vi "ti2.vi"() -> ()   [LabVIEW 2010]
uses:
  typedefs/inspector_state_enum.ctl
  <vilib>/Utility/file.llb/Read From Spreadsheet File (DBL).vi
panel:
  in  "Filter pixels":i32=1 min=1 max=10000 step=1
  in  "Postprocessing":enum32{"Unfiltered", "Filtered"}(radio)
  in  "Channel selection":enum32{"Channel 1", "Channel 2", "Channel 3"}(radio)
  out "Current file":path
  out "Loading":bool
  in  "file path":path
  in  "ZoomOut":bool
  in  "ZoomIn":bool
  in  "Quit":bool
  in  "Load":bool
  out "Overview Graph":cluster{dbl, dbl, "Data out":dbl[]}(graph)
  out "Analysis Graph":dbl[](graph)
  # "Fiber - fMRI\nTrace inspector"
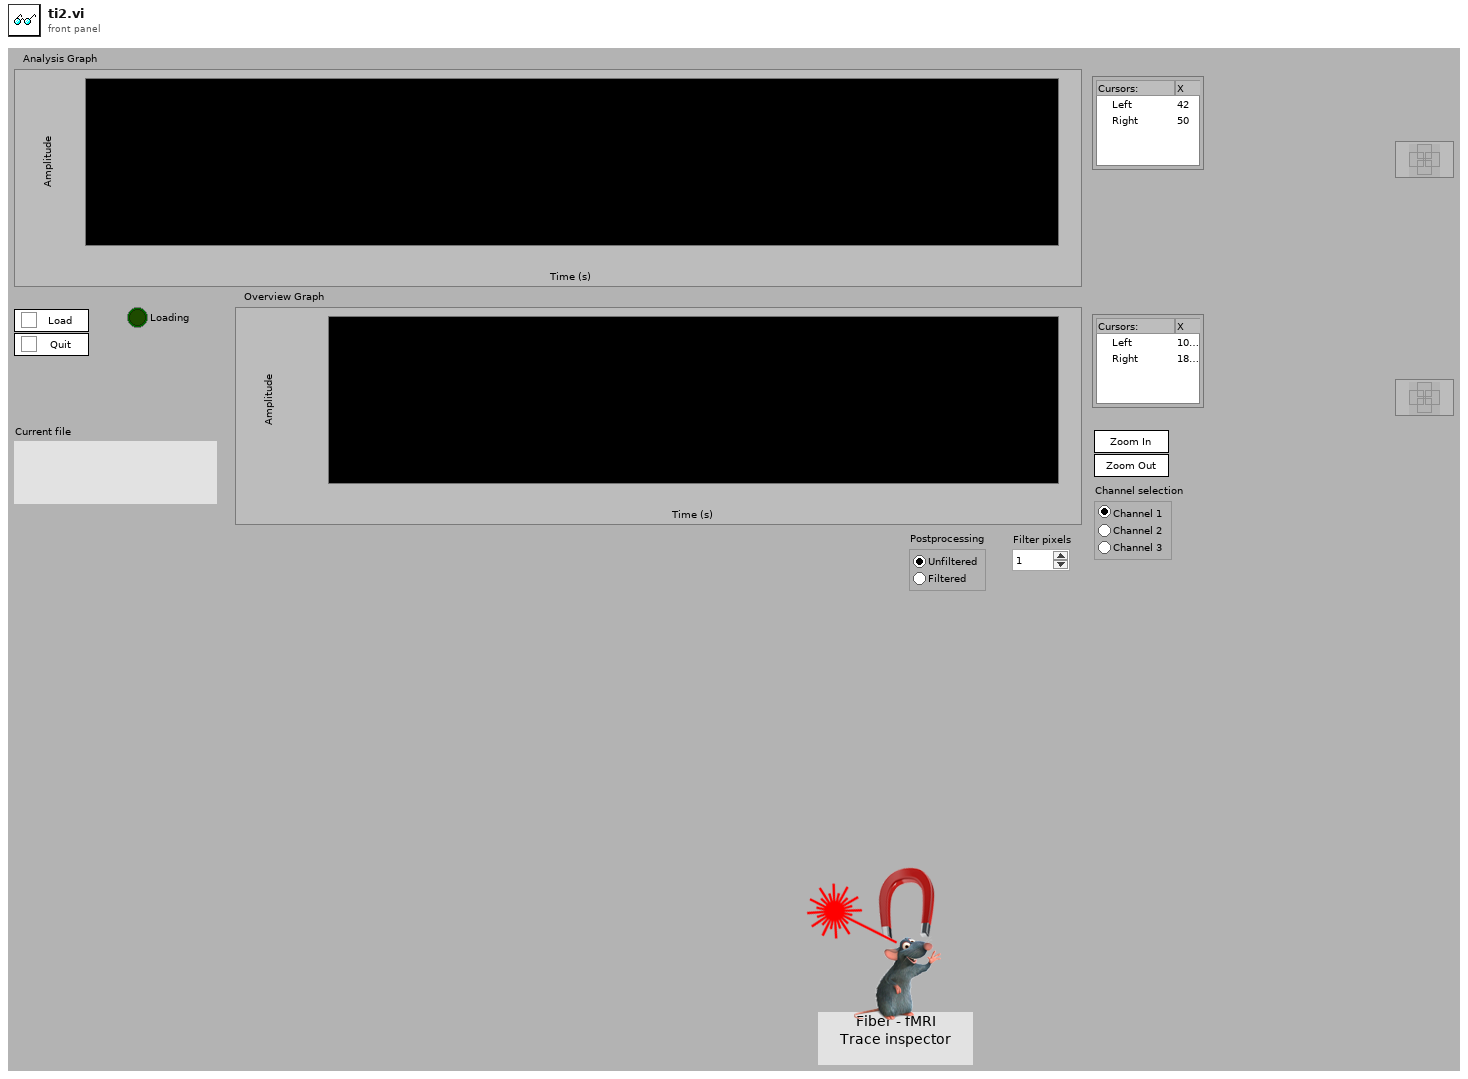
[diagram p1: front panel]
types:
  T1 = typedef "inspector_state_enum.ctl" = enum16{"Init", "Quit", "Error", "ZoomIn", "ZoomOut", "Load", "Update_graphs"}
  T2 = cluster{"Inspector_state_enum":T1, "variant":variant}
  T3 = cluster{"Overview Graph":refnum<vi>, "Analysis Graph":refnum<vi>}
  T4 = cluster{"Channel selection":enum32{"Channel 1", "Channel 2", "Channel 3"}, "Postprocessing":enum32{"Unfiltered", "Filtered"}, "Filter pixels":i32}
  T5 = typedef "LVCursorListTypeDef.ctl" = cluster{"Name":string, "Color":u32, "Style":u8, "Point Style":u8, "Name Visible":bool, "Allow Drag":bool, "Cursor Mode":u32, "Plot":i32, "Index":i32, "Position":cluster{"X":dbl, "Y":dbl}, "X Scale":u32, "Y Scale":u32, "Watch Plots":i32[], "Watch All Plots":bool, "Plot Area":i32, "Label Offset":cluster{"X":dbl, "Y":dbl}}[]
  T6 = cluster{"Name":string, "Color":u32, "Style":u8, "Point Style":u8, "Name Visible":bool, "Allow Drag":bool, "Cursor Mode":u32, "Plot":i32, "Index":i32, "Position":cluster{"X":dbl, "Y":dbl}, "X Scale":u32, "Y Scale":u32, "Watch Plots":i32[], "Watch All Plots":bool, "Plot Area":i32, "Label Offset":cluster{"X":dbl, "Y":dbl}}
  T7 = cluster{"Inspector_state_enum":T1, "variant":variant}[]
  T8 = cluster{"XScale.Minimum":dbl, "XScale.Maximum":dbl}
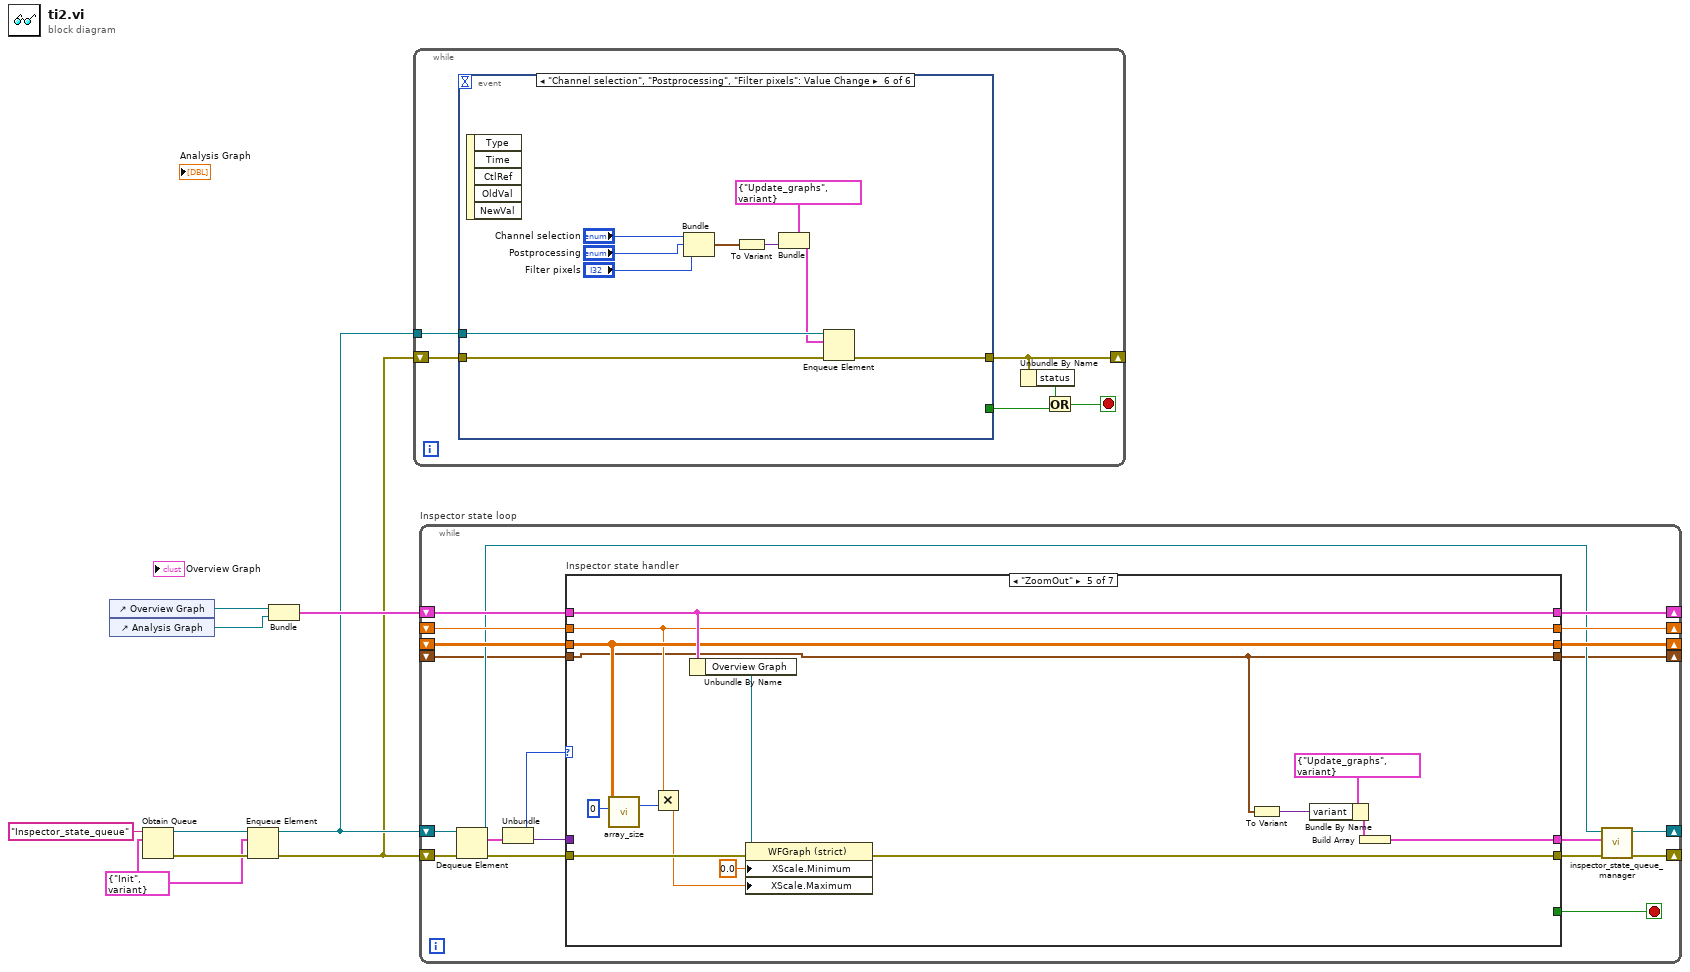
[diagram p0: block diagram]
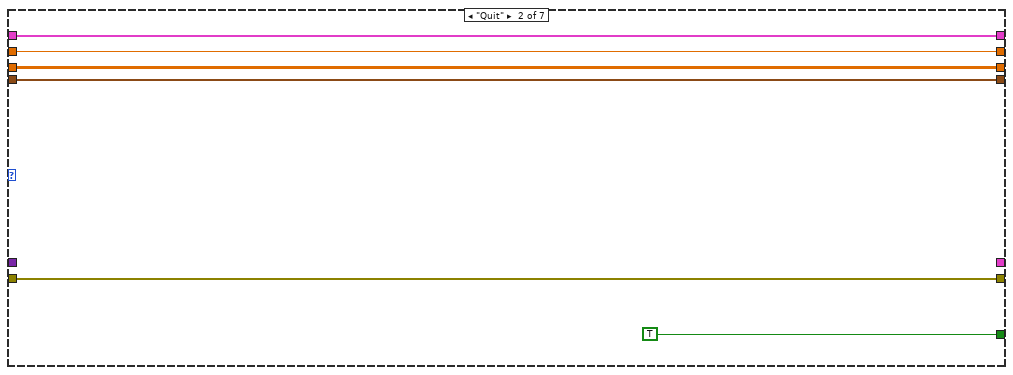
[diagram p3: hidden frame]
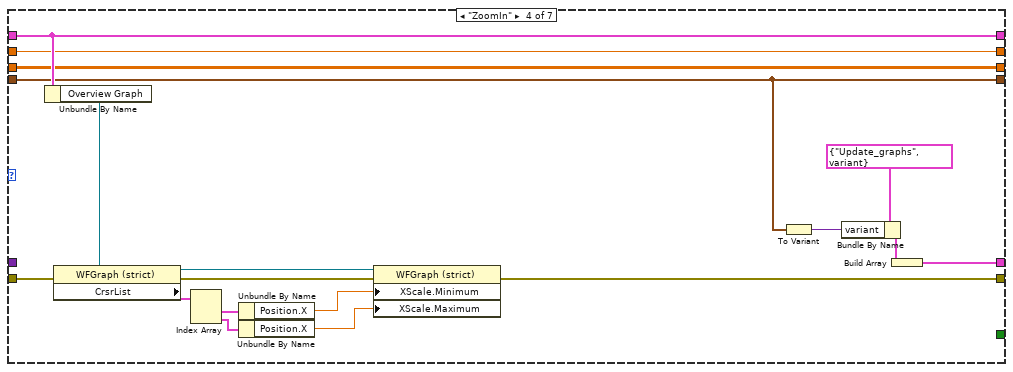
[diagram p5: hidden frame]
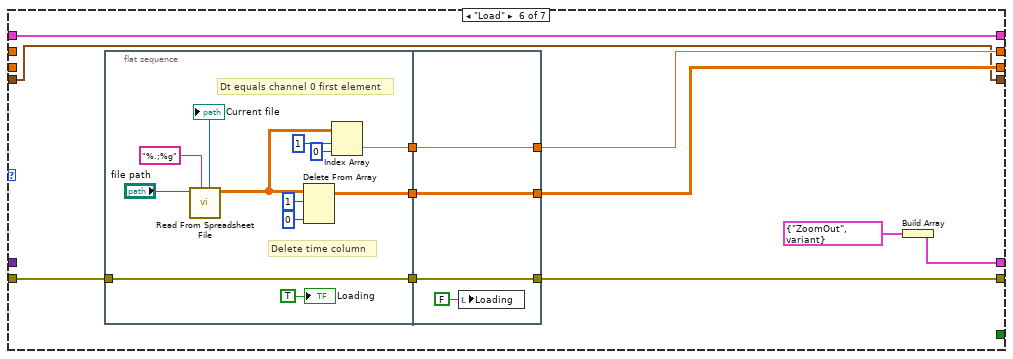
[diagram p6: hidden frame]
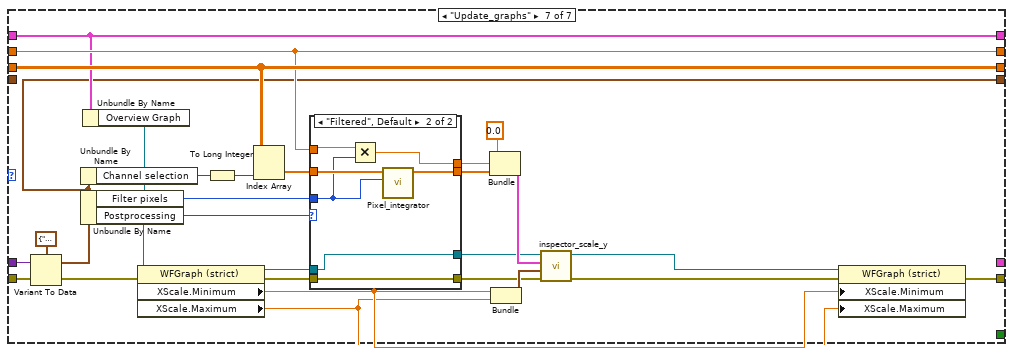
[diagram p7: hidden frame]
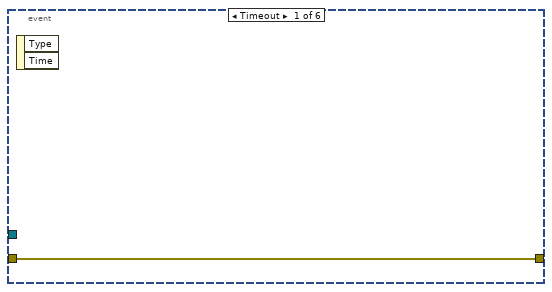
[diagram p9: hidden frame]
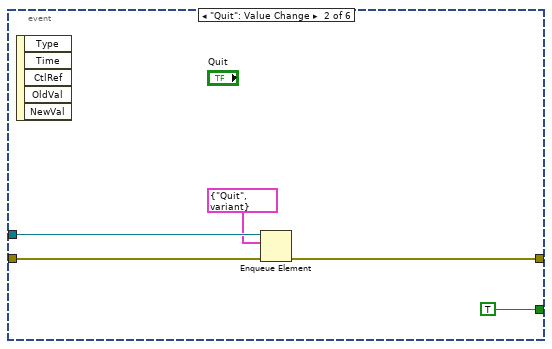
[diagram p10: hidden frame]
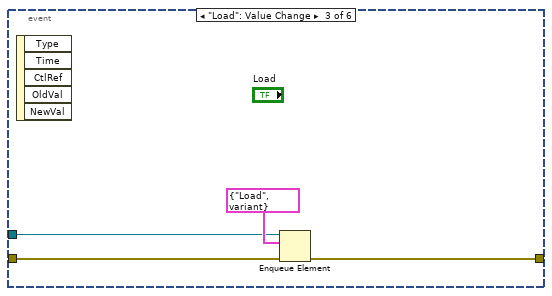
[diagram p11: hidden frame]
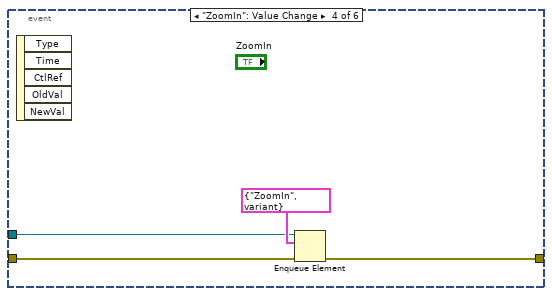
[diagram p12: hidden frame]
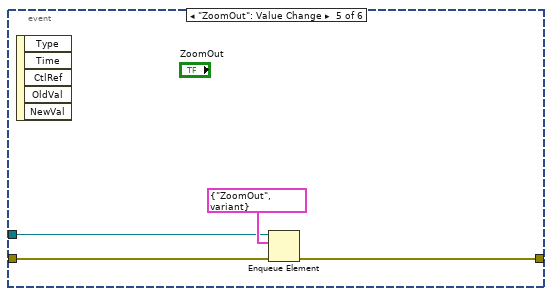
[diagram p13: hidden frame]
diagram:
  w1 = T2 {"Inspector_state_enum"=enum."Init", "variant"=variant}
  n1 = control-ref of="Overview Graph"() -> (w8:refnum<vi>)
  n2 = control-ref of="Analysis Graph"() -> (w7:refnum<vi>)
  n3 = Obtain Queue(name (unnamed)="Inspector_state_queue", element data type=w1) -> (queue out=w5:refnum<queue>, error out=w3:errorcluster)  [unwired: 3 in, 1 out]
  n4 = Enqueue Element(queue=w5, element=w1, error in (no error)=w3) -> (queue out=w4:refnum<queue>, error out=w2:errorcluster)  [unwired: 1 in, 1 out]
  n5 = Bundle("Overview Graph"=w8, "Analysis Graph"=w7) -> (w6:T3)  [unwired: 1 in]
  n6 = while {
    tunnel: w4 -> [w10]
    shift-right: [w14] -> _
    shift-left: w2 -> [w15]
    stop <- w12 stop-if-true
    n7 = event shown="[5] \"Channel selection\", \"Postprocessing\", \"Filter pixels\": Value Change" {
      selector: _ -> [_ _ _ _ _ _]
      dyn-events: _ -> [_ _ _ _ _ _]
      timeout: _ -> [_ _ _ _ _ _]
      tunnel: [w16 w19 w23 w27 w31 w41] -> w14
      tunnel: w15 -> [w16 w20 w24 w28 w32 w42]
      tunnel: [_ TRUE ("y") _ _ _ _] -> w11
      tunnel: w10 -> [_ w18 w22 w26 w30 w43]
      event Timeout {
        n8 = event-data() -> ()  [unwired: 1 in, 2 out]
      }
      event "Quit": Value Change {
        n9 = event-data() -> ()  [unwired: 1 in, 5 out]
        n10 = Enqueue Element(queue=w18, element=T2 {"Inspector_state_enum"=enum."Quit", "variant"=variant}, error in (no error)=w20) -> (error out=w19:errorcluster)  [unwired: 1 in, 2 out]
      }
      event "Load": Value Change {
        n11 = event-data() -> ()  [unwired: 1 in, 5 out]
        n12 = Enqueue Element(queue=w22, element=T2 {"Inspector_state_enum"=enum."Load", "variant"=variant}, error in (no error)=w24) -> (error out=w23:errorcluster)  [unwired: 1 in, 2 out]
      }
      event "ZoomIn": Value Change {
        n13 = event-data() -> ()  [unwired: 1 in, 5 out]
        n14 = Enqueue Element(queue=w26, element=T2 {"Inspector_state_enum"=enum."ZoomIn", "variant"=variant}, error in (no error)=w28) -> (error out=w27:errorcluster)  [unwired: 1 in, 2 out]
      }
      event "ZoomOut": Value Change {
        n15 = event-data() -> ()  [unwired: 1 in, 5 out]
        n16 = Enqueue Element(queue=w30, element=T2 {"Inspector_state_enum"=enum."ZoomOut", "variant"=variant}, error in (no error)=w32) -> (error out=w31:errorcluster)  [unwired: 1 in, 2 out]
      }
      event "Channel selection", "Postprocessing", "Filter pixels": Value Change {
        n17 = event-data() -> ()  [unwired: 1 in, 5 out]
        n18 = Bundle("Channel selection"="Channel selection", "Postprocessing"="Postprocessing", "Filter pixels"="Filter pixels") -> (w36:T4)  [unwired: 1 in]
        n19 = To Variant(anything=w36) -> (Variant=w38:variant)
        n20 = Bundle(cluster=T2 {"Inspector_state_enum"=enum."Update_graphs", "variant"=variant} ("element"), "variant"=w38) -> (w39:T2)  [unwired: 1 in]
        n21 = Enqueue Element(queue=w43, element=w39, error in (no error)=w42) -> (error out=w41:errorcluster)  [unwired: 1 in, 2 out]
      }
    }
    n22 = Unbundle By Name(w14) -> ("status"=w13:bool)
    n23 = Or(x=w13, y=w11) -> (x .or. y?=w12:bool)
  }
  n24 = while "Inspector state loop" {
    shift-right: [w47] -> _
    shift-left: w4 -> [w62]
    shift-right: [w49] -> _
    shift-left: w2 -> [w63]
    shift-right: [w57] -> _
    shift-left: w6 -> [w58]
    shift-right: [w56] -> _
    shift-left: _ -> [w54]
    shift-right: [w55] -> _
    shift-left: _ -> [w53]
    shift-right: [w45] -> _
    shift-left: _ -> [w44]
    stop <- w50 stop-if-true
    n25 = Dequeue Element(queue=w62, error in (no error)=w63) -> (queue out=w48:refnum<queue>, element=w60:T2, error out=w61:errorcluster)  [unwired: 1 in, 1 out]
    n26 = Unbundle(w60) -> ("Inspector_state_enum"=w59:T1, "variant"=w52:variant)
    n27 = case "Inspector state handler" shown="\"ZoomOut\"" w59 {
      tunnel: w61 -> [w68 w74 w79 w96 w110 w120 w167]
      tunnel: [w68 w74 w79 w87 w109 w118 w152] -> w51
      tunnel: [_ TRUE ("y") _ _ _ _ _] -> w50
      tunnel: w58 -> [w67 w72 w78 w97 w112 w123 w155]
      tunnel: [w67 w72 w78 w97 w112 w123 w155] -> w57
      tunnel: [w66 w71 w77 w91 w105 w117 w158] -> w56
      tunnel: [w65 w70 w76 w90 w107 w116 w165] -> w55
      tunnel: w54 -> [w66 w71 w77 w91 w105 _ w158]
      tunnel: w53 -> [w65 w70 w76 w90 w107 _ w165]
      tunnel: w52 -> [_ _ _ _ _ _ w166]
      tunnel: [_ _ _ w84 w100 w115 _] -> w46
      tunnel: [w64 w69 w75 w81 w99 w113 w140] -> w45
      tunnel: w44 -> [w64 w69 w75 w81 w99 w113 _]
      frame "Init", Default {
      }
      frame "Quit" {
      }
      frame "Error" {
      }
      frame "ZoomIn" {
        n28 = Unbundle By Name(w97) -> ("Overview Graph"=w92:refnum<vi>)
        n29 = property class="WFGraph (strict)"(reference=w92, error in=w96) -> (reference out=w89:refnum<vi>, error out=w88:errorcluster, "CrsrList"=w95:T5)
        n30 = Index Array(array=w95) -> (element #1=w94:T6, element #2=w93:T6)  [unwired: 2 in]
        n31 = Unbundle By Name(w94) -> ("Position.X"=w86:dbl)
        n32 = Unbundle By Name(w93) -> ("Position.X"=w85:dbl)
        n33 = property class="WFGraph (strict)"(reference=w89, error in=w88, "XScale.Minimum"=w86, "XScale.Maximum"=w85) -> (error out=w87:errorcluster)  [unwired: 1 out]
        n34 = To Variant(anything=w81) -> (Variant=w82:variant)
        n35 = Bundle By Name(cluster=T2 {"Inspector_state_enum"=enum."Update_graphs", "variant"=variant}, "variant"=w82) -> (w80:T2)
        n36 = Build Array(w80) -> (w84:T7)
      }
      frame "ZoomOut" {
        n37 = call "array_size.vi"("Array"=w107, "Dimension"=0) -> ("Dimension size"=w104:i32)  [unwired: 4 in]
        n38 = Multiply(x=w105, y=w104) -> (x*y=w103:dbl)
        n39 = Unbundle By Name(w112) -> ("Overview Graph"=w111:refnum<vi>)
        n40 = property class="WFGraph (strict)"(reference=w111, error in=w110, "XScale.Minimum"=0.0 ("X Scale.Range:Minimum"), "XScale.Maximum"=w103) -> (error out=w109:errorcluster)  [unwired: 1 out]
        n41 = To Variant(anything=w99) -> (Variant=w102:variant)
        n42 = Bundle By Name(cluster=T2 {"Inspector_state_enum"=enum."Update_graphs", "variant"=variant}, "variant"=w102) -> (w101:T2)
        n43 = Build Array(w101) -> (w100:T7)
      }
      frame "Load" {
        n44 = flat-sequence {
          tunnel: [w125] -> w122
          tunnel: [w132] -> w121
          tunnel: w120 -> [w129]
          tunnel: [w129] -> w119
          tunnel: [w138] -> w117
          tunnel: [w139] -> w116
          tunnel: w122 -> [w139]
          tunnel: w121 -> [w138]
          tunnel: w119 -> [w136]
          tunnel: [w136] -> w118
          frame #0 {
            # "Delete time column"
            # "Dt equals channel 0 first element"
            n45 = call-poly <vilib>:"Read From Spreadsheet File.vi"("format (%.3f)"="%.;%g", "file path (dialog if empty)"="file path") -> ("all rows"=w128:dbl[][], "new file path (Not A Path if cancelled)"=→"Current file":path)  [unwired: 5 in, 3 out]
            n46 = Delete From Array(array=w128, length=1, index (col)=0 ("disabled index (col)")) -> (array with subset deleted=w125:dbl[][])  [unwired: 1 in, 1 out]
            n47 = Index Array(array=w128, index (row)=1 ("disabled index (row)"), index (col)=0 ("disabled index (col)")) -> (element=w132:dbl)
            "Loading" <- TRUE ("Loading")
          }
          frame #1 {
            n48 = local write "Loading"(FALSE ("Loading")) -> ()
          }
        }
        n49 = Build Array(T2 {"Inspector_state_enum"=enum."ZoomOut", "variant"=variant}) -> (w115:T7)
      }
      frame "Update_graphs" {
        n50 = Variant To Data(error in=w167, Variant=w166, type=T4 {"Channel selection"=enum."Channel 1", "Postprocessing"=enum."Unfiltered", "Filter pixels"=0} ("output cluster")) -> (error out=w154:errorcluster, data=w140:T4)
        n51 = Unbundle By Name(w140) -> ("Channel selection"=w162:enum32{"Channel 1", "Channel 2", "Channel 3"})
        n52 = Unbundle By Name(w140) -> ("Filter pixels"=w160:i32, "Postprocessing"=w161:enum32{"Unfiltered", "Filtered"})
        n53 = Unbundle By Name(w155) -> ("Overview Graph"=w153:refnum<vi>)
        n54 = property class="WFGraph (strict)"(reference=w153, error in=w154) -> (reference out=w142:refnum<vi>, error out=w144:errorcluster, "XScale.Minimum"=w147:dbl, "XScale.Maximum"=w146:dbl)
        n55 = To Long Integer(number=w162) -> (32bit integer=w163:i32)
        n56 = Index Array(array=w165, index (col)=w163) -> (element=w159:dbl[])  [unwired: 1 in]
        n57 = case shown="\"Filtered\", Default" w161 {
          tunnel: [w171 w177] -> w148
          tunnel: w159 -> [w171 w178]
          tunnel: w160 -> [_ w175]
          tunnel: w158 -> [w170 w176]
          tunnel: [w170 w174] -> w156
          tunnel: w144 -> [w169 w173]
          tunnel: [w169 w173] -> w143
          tunnel: w142 -> [w168 w172]
          tunnel: [w168 w172] -> w141
          frame "Unfiltered" {
          }
          frame "Filtered", Default {
            n58 = Multiply(x=w176, y=w175) -> (x*y=w174:dbl)
            n59 = call "Pixel_integrator.vi"("Pixels to integrate"=w175, "Data in"=w178) -> ("Data out"=w177:dbl[])  [unwired: 6 in, 1 out]
          }
        }
        n60 = Bundle(0.0, w156, "Data out"=w148) -> (w149:cluster{dbl, dbl, "Data out":dbl[]})  [unwired: 1 in]
        n61 = Bundle("XScale.Minimum"=w147, "XScale.Maximum"=w146) -> (w145:T8)  [unwired: 1 in]
        n62 = call "inspector_scale_y.vi"("error in"=w143, "Borders"=w145, "Waveform in"=w149, "Overview Graph in"=w141) -> ("error out"=w151:errorcluster, "Overview Graph out"=w150:refnum<vi>)  [unwired: 5 in]
        n63 = property class="WFGraph (strict)"(reference=w150, error in=w151, "XScale.Minimum"=w147, "XScale.Maximum"=w146) -> (error out=w152:errorcluster)  [unwired: 1 out]
      }
    }
    n64 = call "inspector_state_queue_manager.vi"("error in"=w51, "State array in"=w46, "Inspector_state_queue in"=w48) -> ("error out"=w49:errorcluster, "Inspector_state_queue out"=w47:refnum<queue>)  [unwired: 7 in]
  }
